vi "Get Value from Database.vi"(8 "error in (no error)":errorcluster, 10 "Entry Name":string, 11 "Message in":refnum<class "String Database.lvclass">=refnum) -> (0 "error out":errorcluster, 1 "Entry Found":bool, 2 "Entry Value":string, 3 "Message out":refnum<class "String Database.lvclass">)   [LabVIEW 2018, in "String Database.lvlib" / "String Database.lvclass"]
uses:
  String Database.lvclass
  String Database.lvclass/String Database.ctl
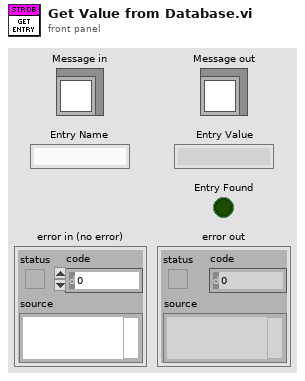
[diagram p1: front panel]
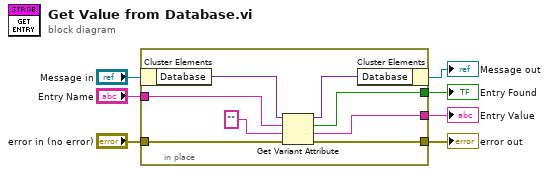
[diagram p0: block diagram]
diagram:
  n1 = in-place {
    in-place-border: "error in (no error)" -> [w15]
    in-place-border: [w14] -> w6
    in-place-border: "Entry Name" -> [w13]
    in-place-border: [w12] -> w4
    in-place-border: [w11] -> w3
    n2 = in-place-cluster #1("Message in") -> ("Database"=w9:variant)
    n3 = Get Variant Attribute(Variant=w9, name=w13, default value (empty Variant)="", error in=w15) -> (duplicate Variant=w8:variant, found=w11:bool, value=w12:string, error out=w14:errorcluster)
    n4 = in-place-cluster #1("Database"=w8) -> (→"Message out":refnum<class "String Database.lvclass">)
  }
  "error out" <- w6
  "Entry Value" <- w4
  "Entry Found" <- w3
